vi "cw_2_7.vi"() -> ()   [LabVIEW 2022 SP3]
panel:
  in  "stop":bool
  out "elapsed time [ms]":dbl
  in  "reset timer":bool
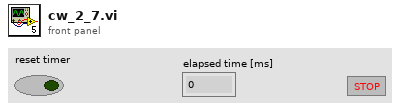
[diagram p1: front panel]
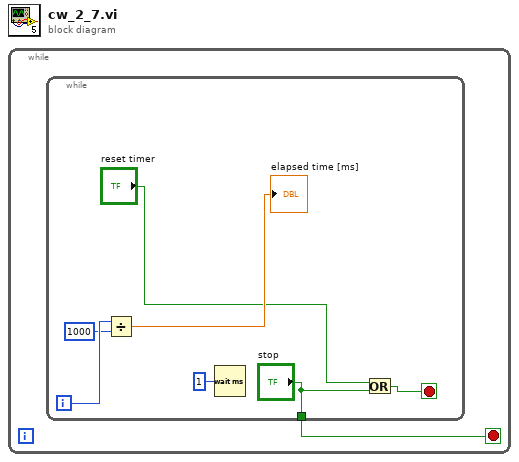
[diagram p0: block diagram]
diagram:
  n1 = while {
    stop <- w1 stop-if-true
    n2 = while {
      tunnel: ["stop"] -> w1
      i -> [w7]
      stop <- w3 stop-if-true
      n3 = Divide(x=w7, y=1000) -> (x/y=→"elapsed time [ms]":dbl)
      n4 = Wait (ms)(milliseconds to wait=u32 1) -> ()  [unwired: 1 out]
      n5 = Or(x="reset timer", y="stop") -> (x .or. y?=w3:bool)
    }
  }
